vi "SynapseAPI-Set Mode.vi"(0 "URL":string="http://localhost:24414", 7 "mode":T1, 11 "error in (no error)":errorcluster) -> (15 "error out":errorcluster)   [LabVIEW 2020]
uses:
  SynapseAPI-Mode.ctl
  <vilib>/httpClient/PUTBuffer.vi
  <vilib>/httpClient/LabVIEWHTTPClient.lvlib
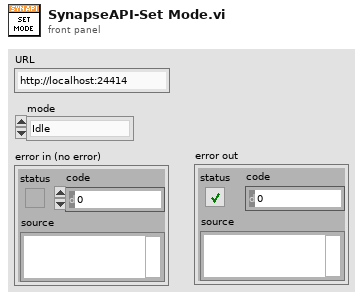
[diagram p1: front panel]
types:
  T1 = typedef "SynapseAPI-Mode.ctl" = enum16{"Idle", "Standby", "Preview", "Record"}
  T2 = typedef "LabVIEWHTTPClient.lvlib/ClientHandle.ctl" = refnum<k1>
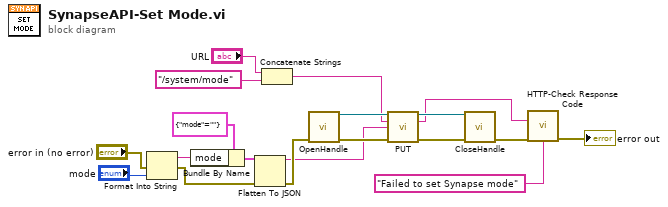
[diagram p0: block diagram]
diagram:
  n1 = Format Into String(error in="error in (no error)", "mode") -> (resulting string=w7:string, error out=w6:errorcluster)  [unwired: 2 in]
  n2 = Bundle By Name(cluster=cluster{"mode":string} {"mode"=""} ("Cluster"), "mode"=w7) -> (w18:cluster{"mode":string})
  n3 = Flatten To JSON(anything=w18, error in (no error)=w6) -> (JSON string=w9:string, 11:w10:errorcluster)  [unwired: 1 in]
  n4 = Concatenate Strings("URL", "/system/mode") -> (w11:string)
  n5 = call <vilib>:"OpenHandle.vi"("error in (no error)"=w10) -> ("client handle out"=w14:T2, "error out"=w13:errorcluster)  [unwired: 13 in]
  n6 = call-poly <vilib>:"PUT.vi"("client handle"=w14, "url"=w11, "buffer"=w9, "error in (no error)"=w13) -> ("client handle out"=w16:T2, "headers"=w2:string, "error out"=w17:errorcluster)  [unwired: 8 in, 1 out]
  n7 = call <vilib>:"CloseHandle.vi"("client handle"=w16, "error in (no error)"=w17) -> ("error out"=w4:errorcluster)  [unwired: 13 in]
  n8 = call "HTTP-Check Response Code.vi"("headers"=w2, "error in"=w4, "message"="Failed to set Synapse mode" ("source")) -> ("error out"=→"error out":errorcluster)  [unwired: 12 in]
